vi "Get Server State UE.vi"(11 "Template Server in":refnum<class "HVC9.lvclass">) -> (2 "Server Internal State UE":refnum<user-event>, 3 "Template Server out":refnum<class "HVC9.lvclass">)   [LabVIEW 2019, in "HVC9.lvlib" / "HVC9.lvclass"]
uses:
  HVC9.lvclass
  typeDefs/Server State Data.ctl
  HVC9.lvclass/HVC9.ctl
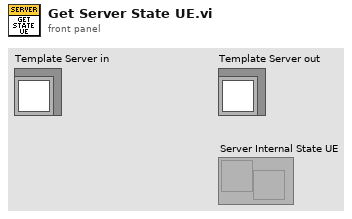
[diagram p1: front panel]
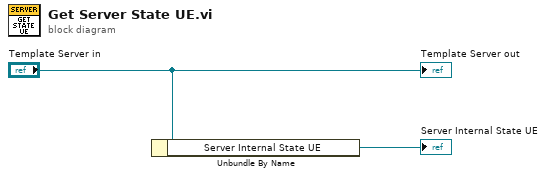
[diagram p0: block diagram]
diagram:
  n1 = Unbundle By Name("Template Server in") -> ("Server Internal State UE"=→"Server Internal State UE":refnum<user-event>)
  "Template Server out" <- "Template Server in"
